vi "_시리얼 포트-초기화.vi"(4 "baud rate":u32=9600 caption="보 전송속도", 5 "시리얼 포트":refnum<visa-resource-name>="COM3") -> (1 "시리얼 포트 2":refnum<visa-resource-name>="COM3", 2 "정상":bool)   [LabVIEW 2015]
uses:
  <vilib>/Instr/_visa.llb/VISA Configure Serial Port (Instr).vi
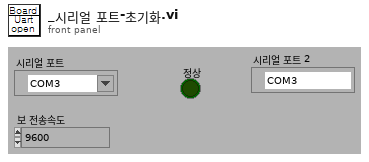
[diagram p1: front panel]
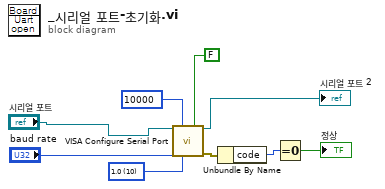
[diagram p0: block diagram]
diagram:
  w6 = u16 10 items=["1.0"=10, "1.5"=15, "2.0"=20] ("stop bits (10: 1 bit)")
  n1 = call-poly "VISA Configure Serial Port"("VISA resource name"="시리얼 포트", "timeout (10sec)"=u32 10000, "Enable Termination\nChar (T)"=FALSE ("Enable Termination\nChar (T)"), "baud rate (9600)"="baud rate", "stop bits (10: 1 bit)"=w6) -> ("VISA resource name out"=→"시리얼 포트 2":refnum<visa-resource-name>, "error out"=w8:errorcluster)  [unwired: 4 in, 5 out]
  n2 = Unbundle By Name(w8) -> ("code"=w7:i32)
  n3 = Equal To 0?(x=w7) -> (x = 0?=→"정상":bool)
